vi "CryoServer Configure.vi"(10 "cntrl q":refnum<queue>, 11 "Ch Names":string[](array[string])) -> (3 "Ch Map":map{string, T1}(c390))   [LabVIEW 2021]
uses:
  CryoServer Channel Mapping.ctl
  Subsystems/SS typedef cluster Instrument Command Queue Data.ctl
panel:
  in  "Cancel":bool
  in  "Save":bool
  in  "Remove":bool
  in  "Add":bool
  in  "Logged Channels":i32[](listbox)
  in  "All  Channels":i32[](listbox)
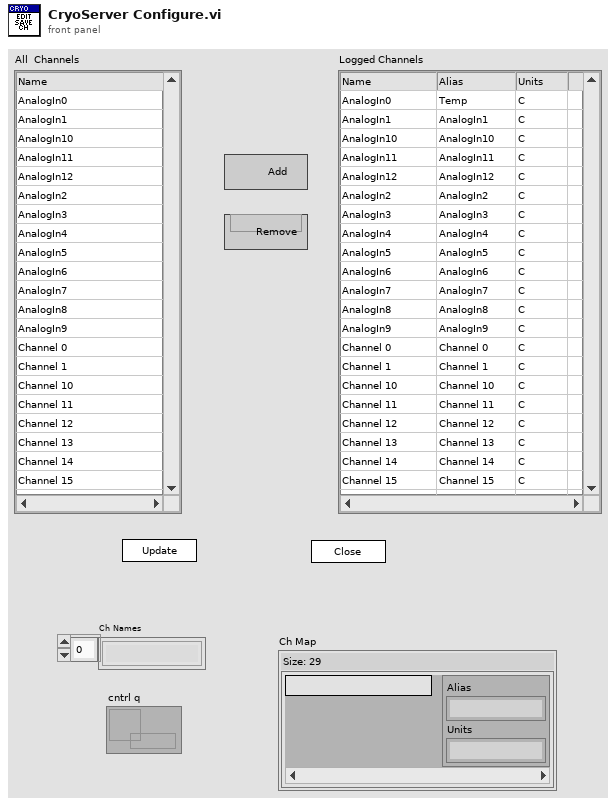
[diagram p1: front panel]
types:
  T1 = typedef "CryoServer Channel Mapping.ctl" = cluster{"Alias":string, "Units":string}
  T2 = cluster{"state":refnum<user-event>, "All":string[], "Ch Map":map{string, T1}, "cntrl q":refnum<queue>}
  T3 = typedef "SS typedef cluster Instrument Command Queue Data.ctl" = cluster{"Cmd":string, "Parameters":variant}
  T4 = typedef "LVRowAndColumnTypeDef.ctl" = cluster{"Row":i32, "Column":i32}
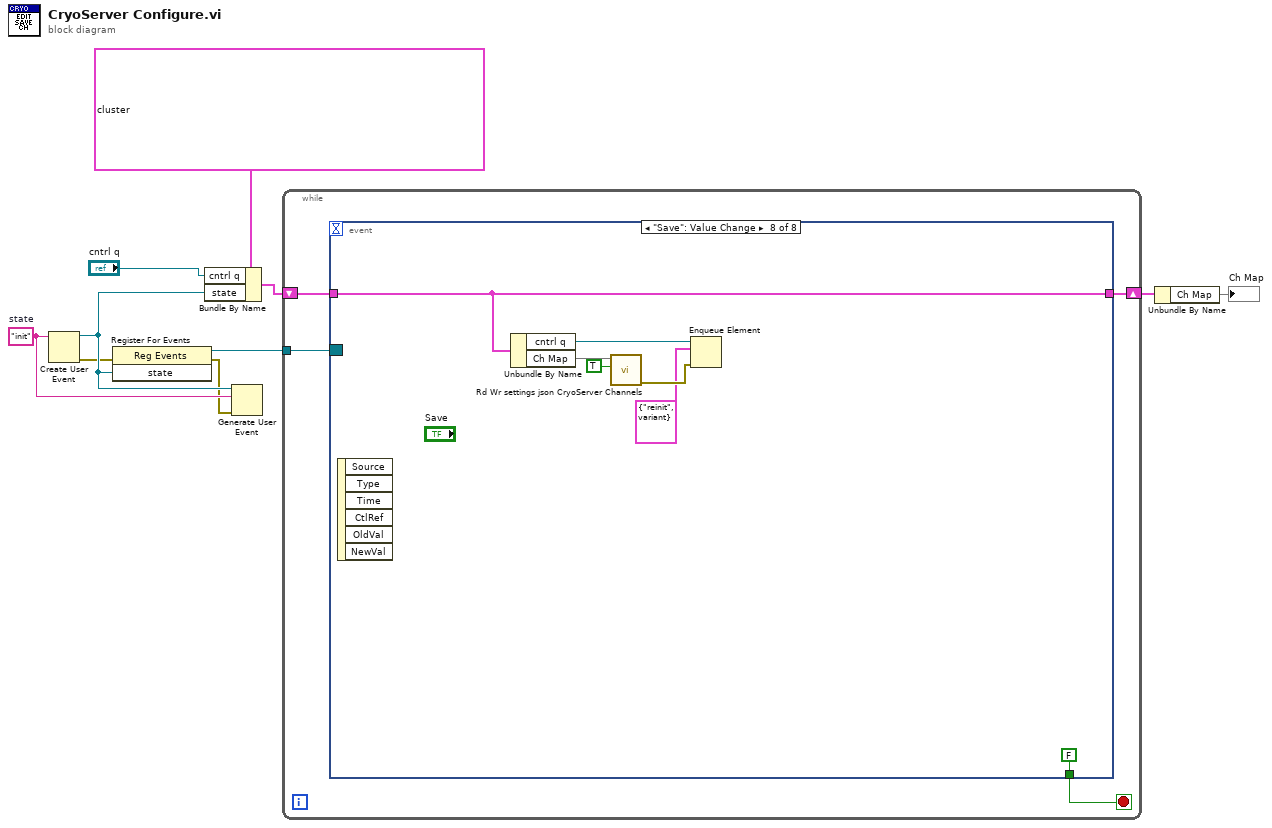
[diagram p0: block diagram]
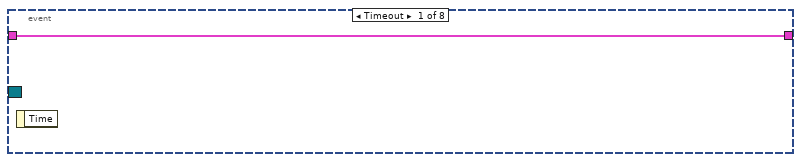
[diagram p2: hidden frame]
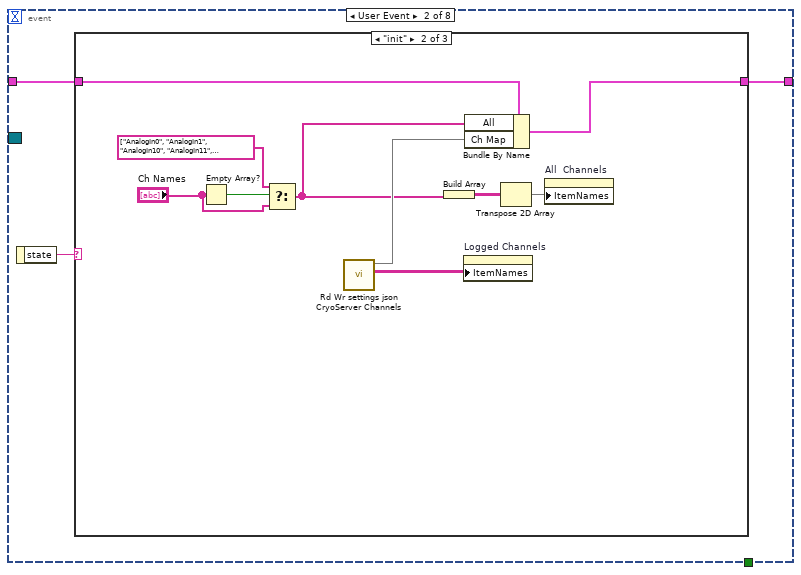
[diagram p3: hidden frame]
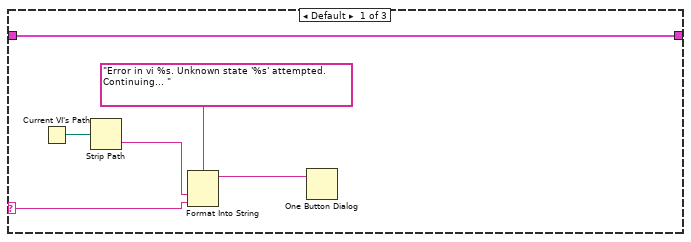
[diagram p4: hidden frame]
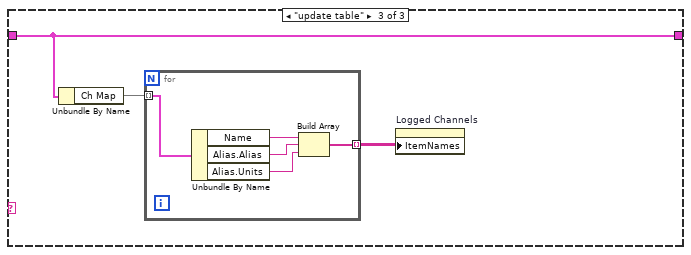
[diagram p5: hidden frame]
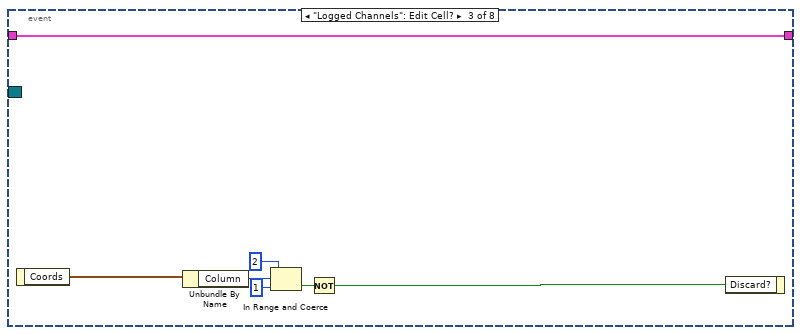
[diagram p6: hidden frame]
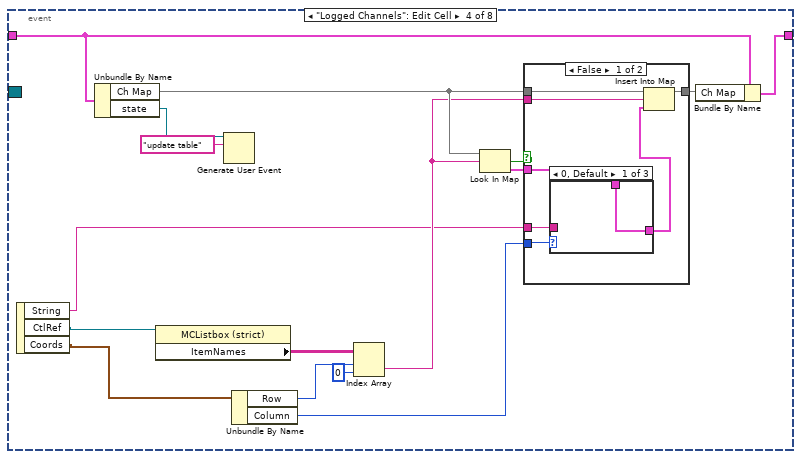
[diagram p7: hidden frame]
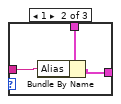
[diagram p8: hidden frame]
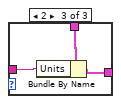
[diagram p9: hidden frame]
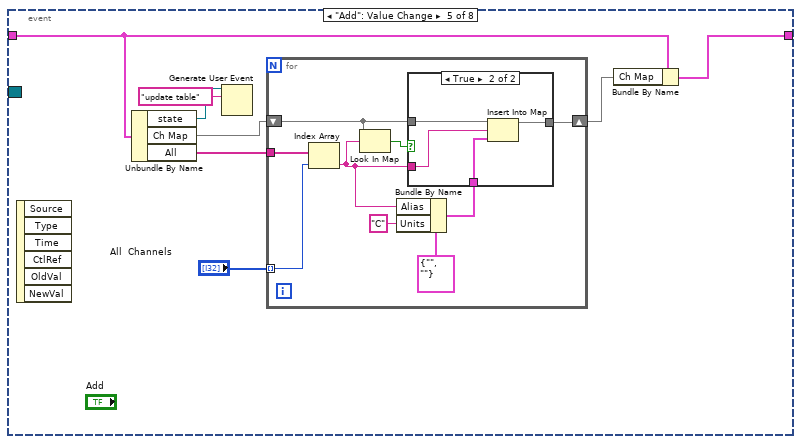
[diagram p11: hidden frame]
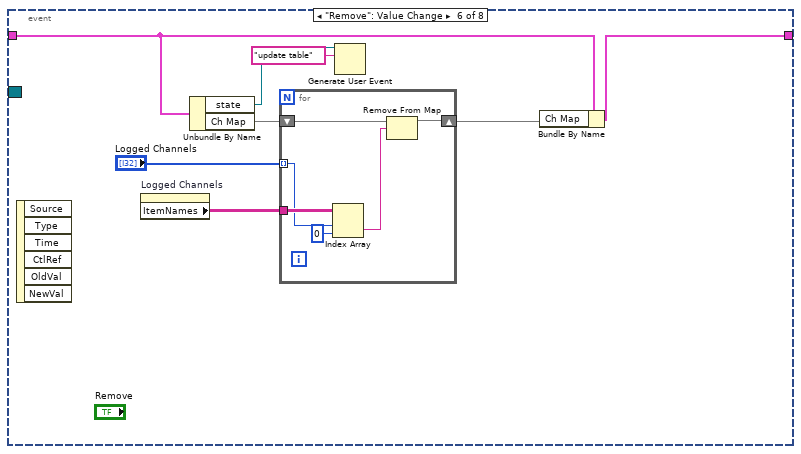
[diagram p13: hidden frame]
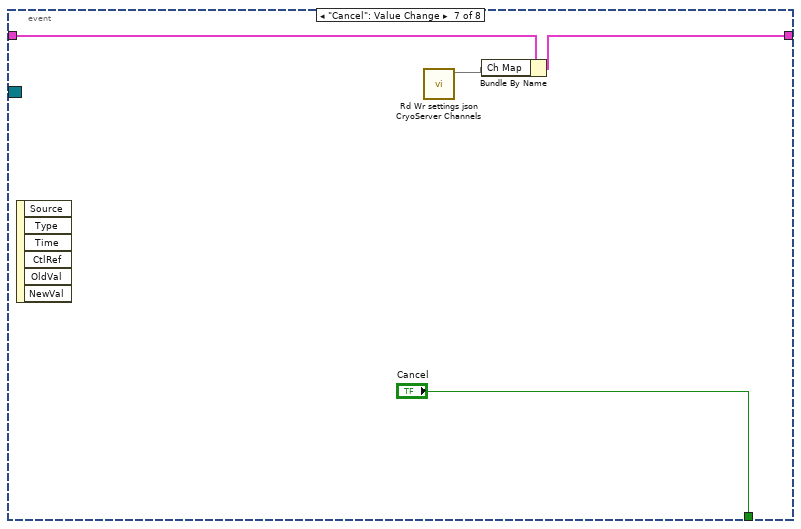
[diagram p14: hidden frame]
diagram:
  w6 = "init"  # state
  n1 = Create User Event(user event datatype=w6) -> (user event=w8:refnum<user-event>, error out=w4:errorcluster)  [unwired: 1 in]
  n2 = register-events(error in=w4, w8) -> (reference out=w7:refnum<event-registration>, error out=w5:errorcluster)  [unwired: 1 in]
  n3 = Bundle By Name(cluster=T2 {"state"=refnum, "All"=["AnalogIn0", "AnalogIn1", "AnalogIn10", "AnalogIn11", "AnalogIn12", "AnalogIn2", "AnalogIn3", "AnalogIn4", "AnalogIn5", "AnalogIn6", "AnalogIn7", "AnalogIn8", "AnalogIn9", "Channel 0", "Channel 1", "Channel 10", "Channel 11", "Channel 12", "Channel 13", "Channel 14", "Channel 15", "Channel 2", "Channel 3", "Channel 4", "Channel 5", "Channel 6", "Channel 7", "Channel 8", "Channel 9", "Coil I Sense (avg)", "CoilVMon", "TimeSecondsSince1970", "UBCFrameNumber0", "aDac", "aDac0", "aDac1", "aDac10", "aDac11", "aDac12", "aDac13", "aDac14", "aDac15", "aDac2", "aDac3", "aDac4", "aDac5", "aDac6", "aDac7", "aDac8", "aDac9", "aDacRaw", "adcCounts", "adcCounts0", "adcCounts1", "adcCounts10", "adcCounts11", "adcCounts12", "adcCounts13", "adcCounts14", "adcCounts15", "adcCounts16", "adcCounts17", "adcCounts18", "adcCounts19", "adcCounts2", "adcCounts20", "adcCounts21", "adcCounts22", "adcCounts23", "adcCounts24", "adcCounts25", "adcCounts26", "adcCounts27", "adcCounts28", "adcCounts29", "adcCounts3", "adcCounts30", "adcCounts31", "adcCounts4", "adcCounts5", "adcCounts6", "adcCounts7", "adcCounts8", "adcCounts9", "address", "analogIn", "analogInRaw", "boardTemp", "boardTempRaw", "coilDAC0", "coilDAC1", "coilDAC2", "coilDAC3", "coilDAC4", "coilDAC5", "coilDAC6", "coilDAC7", "coilDACRaw0", "coilDACRaw1", "coilDACRaw2", "coilDACRaw3", "coilDACRaw4", "coilDACRaw5", "coilDACRaw6", "coilDACRaw7", "coilIsense0", "coilIsense1", "coilIsense2", "coilIsense3", "coilIsense4", "coilIsense5", "coilIsense6", "coilIsense7", "coilIsenseRaw0", "coilIsenseRaw1", "coilIsenseRaw2", "coilIsenseRaw3", "coilIsenseRaw4", "coilIsenseRaw5", "coilIsenseRaw6", "coilIsenseRaw7", "coilVMonRaw", "dacCountsOut0", "dacCountsOut1", "dacCountsOut2", "dacCountsOut3", "demod0", "demod1", "demod10", "demod11", "demod12", "demod13", "demod14", "demod15", "demod2", "demod3", "demod4", "demod5", "demod6", "demod7", "demod8", "demod9", "demodRaw0", "demodRaw1", "demodRaw10", "demodRaw11", "demodRaw12", "demodRaw13", "demodRaw14", "demodRaw15", "demodRaw2", "demodRaw3", "demodRaw4", "demodRaw5", "demodRaw6", "demodRaw7", "demodRaw8", "demodRaw9", "dspidTherm[0]", "dspid[0] Raw", "externalTemp", "externalTempRaw", "frameCounter1Hz", "gDac", "gDac0", "gDac1", "gDac10", "gDac11", "gDac12", "gDac13", "gDac14", "gDac15", "gDac2", "gDac3", "gDac4", "gDac5", "gDac6", "gDac7", "gDac8", "gDac9", "gain", "gnd", "gndRaw", "nsum", "numberOfChannels", "pICFrameCount", "pidAccumulator", "pidError", "pidI", "pidP", "pidSetPoint", "pidSetPointRaw", "readTimeSecondsSince1970", "samplesPerChannel", "status", "syncFrameNumber", "systemNumber", "temperature1", "temperature2", "temperature3", "temperature4", "temperature5", "temperature6", "temperature7", "volts", "volts13", "volts14", "volts15", "volts16", "volts17", "volts18", "volts19", "volts20", "volts21", "volts22", "volts23", "volts24", "volts25", "volts26", "volts27", "volts28", "volts29", "volts30", "volts31", "voltsOut0", "voltsOut1", "voltsOut2", "voltsOut3", "vsupply", "vsupplyRaw"], "Ch Map"={}, "cntrl q"=refnum}, "cntrl q"="cntrl q", "state"=w8) -> (w9:T2)
  n4 = Generate User Event(user event=w8, event data cluster=w6, error in=w5) -> ()  [unwired: 1 in, 2 out]
  n5 = while {
    tunnel: w7 -> [w14]
    shift-right: [w12] -> w3
    shift-left: w9 -> [w13]
    stop <- w11 stop-if-true
    n6 = event shown="[7] \"Save\": Value Change" {
      selector: w14 -> [_ _ _ _ _ _ _ _]
      dyn-events: _ -> [_ _ _ _ _ _ _ _]
      timeout: _ -> [_ _ _ _ _ _ _ _]
      tunnel: w13 -> [w15 w17 w49 w54 w85 w107 w117 w127]
      tunnel: [w15 w16 w49 w55 w86 w108 w118 w127] -> w12
      tunnel: [_ _ _ _ _ _ "Cancel" FALSE ("Cancel")] -> w11
      event Timeout {
        n7 = event-data() -> ()  [unwired: 1 in, 1 out]
      }
      event User Event {
        n8 = event-data() -> ("state"=w18:string)  [unwired: 1 in]
        n9 = case shown="\"init\"" w18 {
          selector: w18 -> [w23 _ _]
          tunnel: w17 -> [w19 w27 w37]
          tunnel: [w19 w28 w37] -> w16
          frame Default {
            n10 = Current VI's Path() -> (path=w22:path)
            n11 = Strip Path(path=w22) -> (name=w21:string)  [unwired: 1 out]
            n12 = Format Into String(format string="Error in vi %s. Unknown state '%s' attempted. Continuing... ", w21, w23) -> (resulting string=w20:string)  [unwired: 2 in, 1 out]
            n13 = One Button Dialog(message=w20) -> ()  [unwired: 1 in, 1 out]
          }
          frame "init" {
            n14 = Empty Array?(array="Ch Names") -> (empty?=w34:bool)
            n15 = Select(t=string[] ["AnalogIn0", "AnalogIn1", "AnalogIn10", "AnalogIn11", "AnalogIn12", "AnalogIn2", "AnalogIn3", "AnalogIn4", "AnalogIn5", "AnalogIn6", "AnalogIn7", "AnalogIn8", "AnalogIn9", "Channel 0", "Channel 1", "Channel 10", "Channel 11", "Channel 12", "Channel 13", "Channel 14", "Channel 15", "Channel 2", "Channel 3", "Channel 4", "Channel 5", "Channel 6", "Channel 7", "Channel 8", "Channel 9", "Coil I Sense (avg)", "CoilVMon", "TimeSecondsSince1970", "UBCFrameNumber0", "aDac", "aDac0", "aDac1", "aDac10", "aDac11", "aDac12", "aDac13", "aDac14", "aDac15", "aDac2", "aDac3", "aDac4", "aDac5", "aDac6", "aDac7", "aDac8", "aDac9", "aDacRaw", "adcCounts", "adcCounts0", "adcCounts1", "adcCounts10", "adcCounts11", "adcCounts12", "adcCounts13", "adcCounts14", "adcCounts15", "adcCounts16", "adcCounts17", "adcCounts18", "adcCounts19", "adcCounts2", "adcCounts20", "adcCounts21", "adcCounts22", "adcCounts23", "adcCounts24", "adcCounts25", "adcCounts26", "adcCounts27", "adcCounts28", "adcCounts29", "adcCounts3", "adcCounts30", "adcCounts31", "adcCounts4", "adcCounts5", "adcCounts6", "adcCounts7", "adcCounts8", "adcCounts9", "address", "analogIn", "analogInRaw", "boardTemp", "boardTempRaw", "coilDAC0", "coilDAC1", "coilDAC2", "coilDAC3", "coilDAC4", "coilDAC5", "coilDAC6", "coilDAC7", "coilDACRaw0", "coilDACRaw1", "coilDACRaw2", "coilDACRaw3", "coilDACRaw4", "coilDACRaw5", "coilDACRaw6", "coilDACRaw7", "coilIsense0", "coilIsense1", "coilIsense2", "coilIsense3", "coilIsense4", "coilIsense5", "coilIsense6", "coilIsense7", "coilIsenseRaw0", "coilIsenseRaw1", "coilIsenseRaw2", "coilIsenseRaw3", "coilIsenseRaw4", "coilIsenseRaw5", "coilIsenseRaw6", "coilIsenseRaw7", "coilVMonRaw", "dacCountsOut0", "dacCountsOut1", "dacCountsOut2", "dacCountsOut3", "demod0", "demod1", "demod10", "demod11", "demod12", "demod13", "demod14", "demod15", "demod2", "demod3", "demod4", "demod5", "demod6", "demod7", "demod8", "demod9", "demodRaw0", "demodRaw1", "demodRaw10", "demodRaw11", "demodRaw12", "demodRaw13", "demodRaw14", "demodRaw15", "demodRaw2", "demodRaw3", "demodRaw4", "demodRaw5", "demodRaw6", "demodRaw7", "demodRaw8", "demodRaw9", "dspidTherm[0]", "dspid[0] Raw", "externalTemp", "externalTempRaw", "frameCounter1Hz", "gDac", "gDac0", "gDac1", "gDac10", "gDac11", "gDac12", "gDac13", "gDac14", "gDac15", "gDac2", "gDac3", "gDac4", "gDac5", "gDac6", "gDac7", "gDac8", "gDac9", "gain", "gnd", "gndRaw", "nsum", "numberOfChannels", "pICFrameCount", "pidAccumulator", "pidError", "pidI", "pidP", "pidSetPoint", "pidSetPointRaw", "readTimeSecondsSince1970", "samplesPerChannel", "status", "syncFrameNumber", "systemNumber", "temperature1", "temperature2", "temperature3", "temperature4", "temperature5", "temperature6", "temperature7", "volts", "volts13", "volts14", "volts15", "volts16", "volts17", "volts18", "volts19", "volts20", "volts21", "volts22", "volts23", "volts24", "volts25", "volts26", "volts27", "volts28", "volts29", "volts30", "volts31", "voltsOut0", "voltsOut1", "voltsOut2", "voltsOut3", "vsupply", "vsupplyRaw"] ("subarray"), s=w34, f="Ch Names") -> (s? t:f=w26:string[])
            n16 = call "Rd Wr settings json CryoServer Channels.vi"() -> ("Ch Names"=w25:string[][], "CryoServer Channels out"=w29:map{string, T1})  [unwired: 9 in, 1 out]
            n17 = Build Array(w26) -> (w31:string[][])
            n18 = property on="Logged Channels" class="MCListbox (strict)"("ItemNames"=w25) -> ()  [unwired: 2 in, 2 out]
            n19 = Bundle By Name(cluster=w27, "All"=w26, "Ch Map"=w29) -> (w28:T2)
            n20 = Transpose 2D Array(2D array=w31) -> (transposed array=w30:string[][])
            n21 = property on="All  Channels" class="MCListbox (strict)"("ItemNames"=w30) -> ()  [unwired: 2 in, 2 out]
          }
          frame "update table" {
            n22 = Unbundle By Name(w37) -> ("Ch Map"=w36:map{string, T1})
            n23 = for {
              tunnel: w36 -> [w42] mode=indexing
              tunnel: [w38] -> w35 mode=indexing
              n24 = Unbundle By Name(w42) -> ("Name"=w41:string, "Alias.Alias"=w40:string, "Alias.Units"=w39:string)
              n25 = Build Array(w41, w40, w39) -> (w38:string[])
            }
            n26 = property on="Logged Channels" class="MCListbox (strict)"("ItemNames"=w35) -> ()  [unwired: 2 in, 2 out]
          }
        }
      }
      event "Logged Channels": Edit Cell? {
        n27 = event-data() -> ("Coords"=w43:T4)  [unwired: 1 in]
        n28 = Unbundle By Name(w43) -> ("Column"=w48:i32)
        n29 = In Range and Coerce(upper limit=2, x=w48, lower limit=1) -> (In Range?=w45:bool)  [unwired: 1 out]
        n30 = Not(x=w45) -> (.not. x?=w44:bool)
        n31 = event-data("Discard?"=w44) -> ()  [unwired: 1 in, 1 out]
      }
      event "Logged Channels": Edit Cell {
        n32 = event-data() -> ("String"=w57:string, "CtlRef"=w50:refnum<vi>, "Coords"=w51:T4)  [unwired: 1 in]
        n33 = Unbundle By Name(w54) -> ("Ch Map"=w63:map{string, T1}, "state"=w53:refnum<user-event>)
        n34 = property class="MCListbox (strict)"(reference=w50) -> ("ItemNames"=w60:string[][])  [unwired: 1 in, 2 out]
        n35 = Generate User Event(user event=w53, event data cluster="update table" ("event data")) -> ()  [unwired: 2 in, 2 out]
        n36 = Unbundle By Name(w51) -> ("Row"=w65:i32, "Column"=w59:i32)
        n37 = Index Array(array=w60, index (row)=w65, index (col)=0 ("disabled index (col)")) -> (element=w58:string)
        n38 = Look In Map(map=w63, key=w58) -> (key not found?=w62:bool, value=w61:T1)  [unwired: 1 in]
        n39 = case shown="False" w62 {
          tunnel: w63 -> [w72 w80]
          tunnel: w61 -> [w71 _]
          tunnel: w59 -> [w69 _]
          tunnel: w58 -> [w70 _]
          tunnel: w57 -> [w68 _]
          tunnel: [w66 w80] -> w56
          frame False {
            n40 = case shown="0, Default" w69 {
              tunnel: w71 -> [w73 w76 w79]
              tunnel: w68 -> [_ w75 w78]
              tunnel: [w73 w74 w77] -> w67
              frame 0, Default {
              }
              frame 1 {
                n41 = Bundle By Name(cluster=w76, "Alias"=w75) -> (w74:T1)
              }
              frame 2 {
                n42 = Bundle By Name(cluster=w79, "Units"=w78) -> (w77:T1)
              }
            }
            n43 = Insert Into Map(map in=w72, key=w70, value=w67) -> (map out=w66:map{string, T1})  [unwired: 2 out]
          }
          frame True {
          }
        }
        n44 = Bundle By Name(cluster=w54, "Ch Map"=w56) -> (w55:T2)
      }
      event "Add": Value Change {
        n45 = event-data() -> ()  [unwired: 1 in, 6 out]
        n46 = Unbundle By Name(w85) -> ("state"=w82:refnum<user-event>, "Ch Map"=w84:map{string, T1}, "All"=w88:string[])
        n47 = Generate User Event(user event=w82, event data cluster="update table" ("event data")) -> ()  [unwired: 2 in, 2 out]
        n48 = for {
          tunnel: w88 -> [w97]
          tunnel: "All  Channels" -> [w96] mode=indexing
          shift-right: [w95] -> w83
          shift-left: w84 -> [w92]
          n49 = Index Array(array=w97, index=w96) -> (element=w91:string)
          n50 = Look In Map(map=w92, key=w91) -> (key not found?=w93:bool)  [unwired: 1 in, 1 out]
          n51 = Bundle By Name(cluster=T1 {"Alias"="", "Units"=""} ("value"), "Alias"=w91, "Units"="C") -> (w90:T1)
          n52 = case shown="True" w93 {
            tunnel: [w98 w102] -> w95
            tunnel: w92 -> [w98 w101]
            tunnel: w91 -> [_ w100]
            tunnel: w90 -> [_ w99]
            frame False {
            }
            frame True {
              n53 = Insert Into Map(map in=w101, key=w100, value=w99) -> (map out=w102:map{string, T1})  [unwired: 2 out]
            }
          }
        }
        n54 = Bundle By Name(cluster=w85, "Ch Map"=w83) -> (w86:T2)
      }
      event "Remove": Value Change {
        n55 = event-data() -> ()  [unwired: 1 in, 6 out]
        n56 = property on="Logged Channels" class="MCListbox (strict)"() -> ("ItemNames"=w105:string[][])  [unwired: 2 in, 2 out]
        n57 = Unbundle By Name(w107) -> ("state"=w104:refnum<user-event>, "Ch Map"=w110:map{string, T1})
        n58 = for {
          tunnel: "Logged Channels" -> [w115] mode=indexing
          shift-right: [w111] -> w106
          shift-left: w110 -> [w113]
          tunnel: w105 -> [w116]
          n59 = Index Array(array=w116, index (row)=w115, index (col)=0 ("disabled index (col)")) -> (element=w112:string)
          n60 = Remove From Map(10:w112, 11:w113) -> (3:w111:map{string, T1})  [unwired: 2 out]
        }
        n61 = Generate User Event(user event=w104, event data cluster="update table" ("event data")) -> ()  [unwired: 2 in, 2 out]
        n62 = Bundle By Name(cluster=w107, "Ch Map"=w106) -> (w108:T2)
      }
      event "Cancel": Value Change {
        n63 = event-data() -> ()  [unwired: 1 in, 6 out]
        n64 = call "Rd Wr settings json CryoServer Channels.vi"() -> ("CryoServer Channels out"=w119:map{string, T1})  [unwired: 9 in, 2 out]
        n65 = Bundle By Name(cluster=w117, "Ch Map"=w119) -> (w118:T2)
      }
      event "Save": Value Change {
        n66 = event-data() -> ()  [unwired: 1 in, 6 out]
        n67 = Unbundle By Name(w127) -> ("cntrl q"=w123:refnum<queue>, "Ch Map"=w124:map{string, T1})
        n68 = call "Rd Wr settings json CryoServer Channels.vi"("Write? (F:Read)"=TRUE, "CryoServer Channels"=w124) -> ("error out"=w122:errorcluster)  [unwired: 7 in, 2 out]
        n69 = Enqueue Element(queue=w123, element=T3 {"Cmd"="reinit", "Parameters"=variant}, error in (no error)=w122) -> ()  [unwired: 1 in, 3 out]
      }
    }
  }
  n70 = Unbundle By Name(w3) -> ("Ch Map"=→"Ch Map":map{string, T1})
